vi "AnalogCNTL_Dakota2ch.vi"() -> ()   [LabVIEW 2015]
uses:
  <userlib>/caLab/Private/Put_DBL-1D_PV-1D.vi
  <vilib>/addons/control/pid/pid.llb/PID (DBL).vi
  <userlib>/caLab/Private/Get_PV-1D.vi
  <vilib>/addons/control/pid/NI_PID_pid.lvlib
  <vilib>/Analysis/NI_AALPro.lvlib
panel:
  out "slope OK":bool
  in  "slope loop":u8=15 min=10 max=30 step=1
  in  "Inlet2 offset":dbl
  out "APX:CellPressureState":u32
  in  "Threshold":dbl format="%#_13g"
  out "Inlet More":bool
  out "APX:OmniaxZ 2":dbl
  out "Open 2":bool
  in  "Gas_in_min_LIM 2":dbl min=0.0 max=0.3 step=0.02 format="%_3g"
  in  "Gas_in_max_LIM 2":dbl min=0.0 max=2.0 step=0.02 format="%_3g"
  out "Inlet2":dbl(slide) scale=0.3..0.8
  out "APX:CellIn2_Mv":dbl
  out "APX:CellOut_MV":dbl
  out "OmniazZ Failure":bool
  out "APX:CellMode":dbl
  out "APX:OmniaxZ":dbl
  out "APX:CellPressureState_LED":i16(slide) scale=0.0..3.0
  out "APX:CellPressureStateorg":i16
  out "APX:CellMode":bool
  out "PID_P":dbl format="%_4g"
  out "HPC Pressure Failure":bool
  out "HPC Turbo failure":bool
  out "<1.3":bool
  out "<2":bool
  out "APX:V7_SCL":bool
  out "APX:V7_SOP":bool
  out "OpenEx":bool
  out "APX:GAS":dbl format="%.2f"
  out "APX:CellIn_MV":dbl
  out "slope":dbl
  out "Open 1":bool
  in  "Inlet Mode":u16(ring) items=["Close", "Open", "Auto"]
  out "Inlet":sgl(slide)=0.8 min=0.3 max=0.8 step=0.05 scale=0.3..0.8
  out "Status":bool
  out "CellMode":u16
  out "Gas_out_max":dbl
  out "Period":i32
  out "Open Period":i32
  in  "Gas_in_min_LIM":dbl min=0.0 max=0.3 step=0.02 format="%_3g"
  in  "Gain":dbl=1.0 min=1.0 max=50.0 step=1.0 format="%_3g"
  in  "Gas_in_max_LIM":dbl=0.85 min=0.0 max=0.9 step=0.02 format="%_3g"
  in  "PID_D":dbl min=0.0 max=5.0 step=0.02 format="%_3g"
  in  "PID_I":dbl=0.5 min=0.005 max=5.0 step=0.02 format="%_3g"
  in  "PID_P_base":dbl=1.0 min=0.005 max=5.0 step=0.02 format="%_3g"
  in  "APX:CellPressure_RV":dbl=0.05 min=0.001 max=5.0 step=0.001 format="%.3f"
  out "PID_OC":dbl format="%.2f"
  out "PID dt out (s)":dbl format="%.3f"
  out "CellPressure":dbl(graph)
  in  "Exhasuet Mode":u16(ring) items=["Close", "Open", "Auto"]
  out "APX:AP1":dbl format="%#_3g"
  out "Outlet":sgl(slide)=2.0 min=0 max=5 step=0.05 scale=0.0..5.0
  out "APX:HPC":dbl format="%#_3g"
  out "APX:CellPressure_PV":dbl format="%_5g"
  in  "stop":bool
  # "Close-Close"
  # "Close-Open"
  # "Mk-II"
  # "0:Evacuate\n1: Auto-Auto\n2: Man-Man\n3: Man-Auto\n4: Auto-Man"
  # "Dakota 100000 sccm"
  # "if P>0.1 Period=Px100"
  # "8E-7 torr"
  # "record(ao, \"APX:CellIn_RV\")\n{\n    field(DESC, \"Double input without range infos\")\n    field(EGU, \"NA\")\n    field(PINI, \"YES\")\n}\nrecord(ao, \"APX:CellOut_RV\")\n{\n    field(DESC, \"Double input without range infos\")\n    field(EGU, \"NA\")\n    field(PINI, \"YES\")\n}\nrecord(ao, \"APX:CellIn_MV\")\n{\n    field(DESC, \"Double input without range infos\")\n    field(EGU, \"NA\")\n    field(PINI, \"YES\")\n}\nrecord(ao, \"APX:CellOut_MV\")\n{\n    field(DESC, \"Double input without range infos\")\n    field(EGU, \"NA\")\n    field(PINI, \"YES\")"
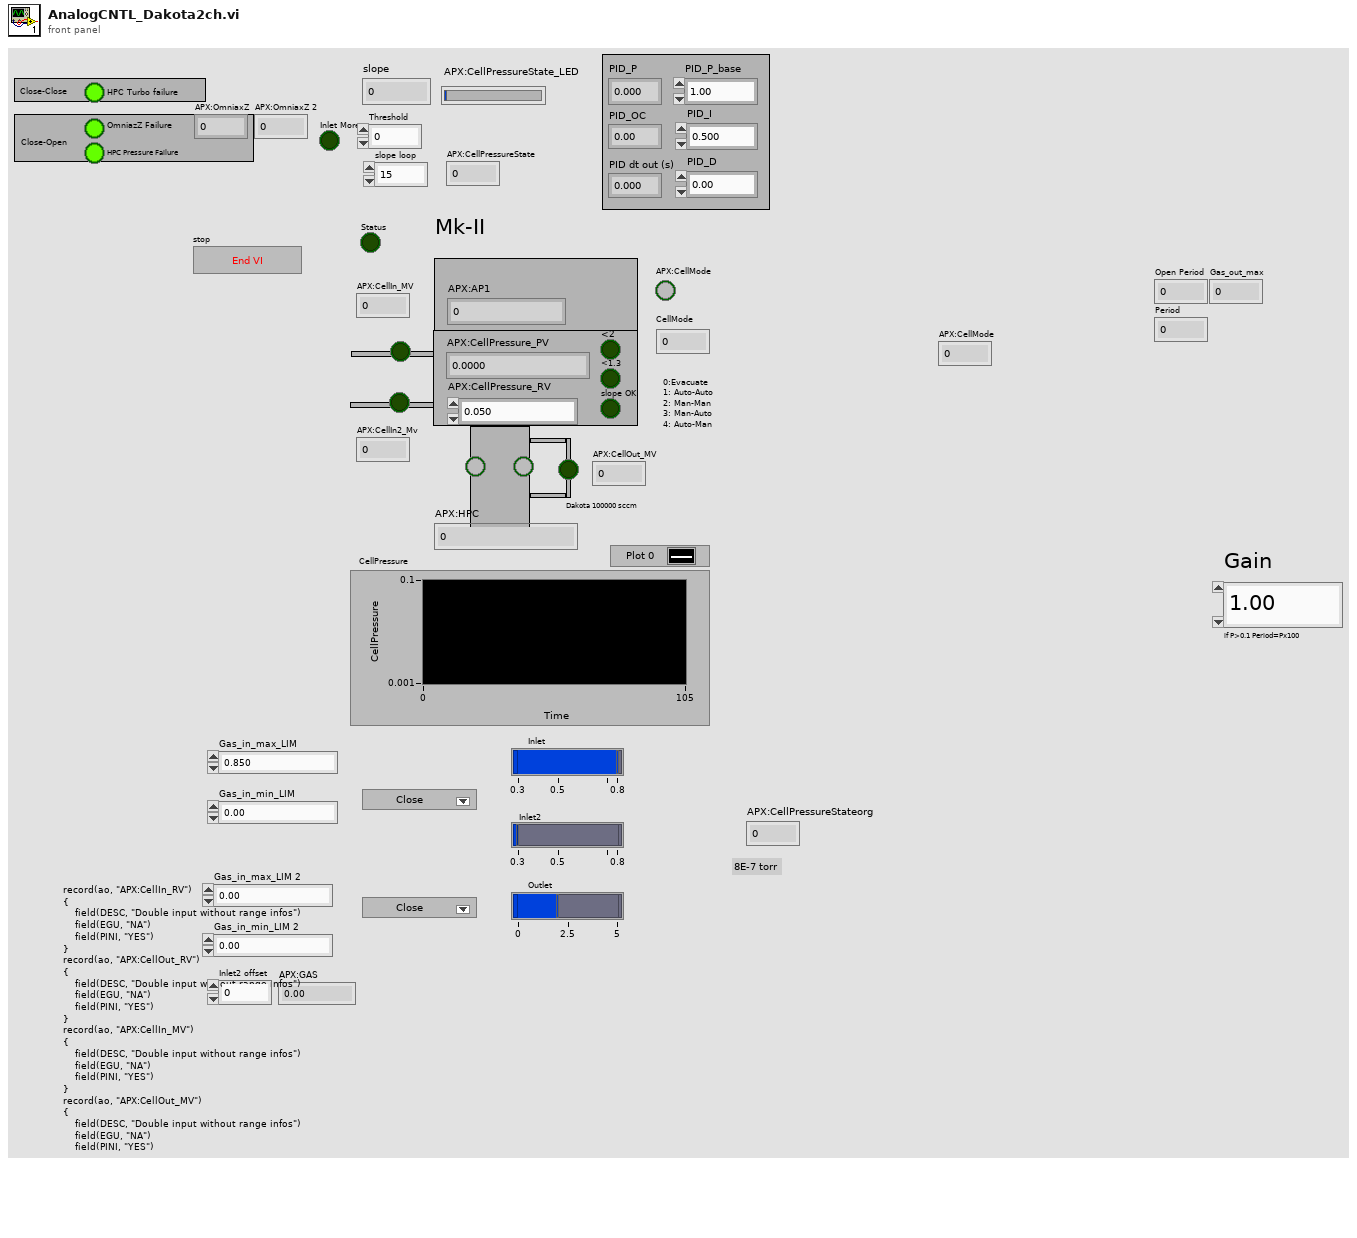
[diagram p1: front panel]
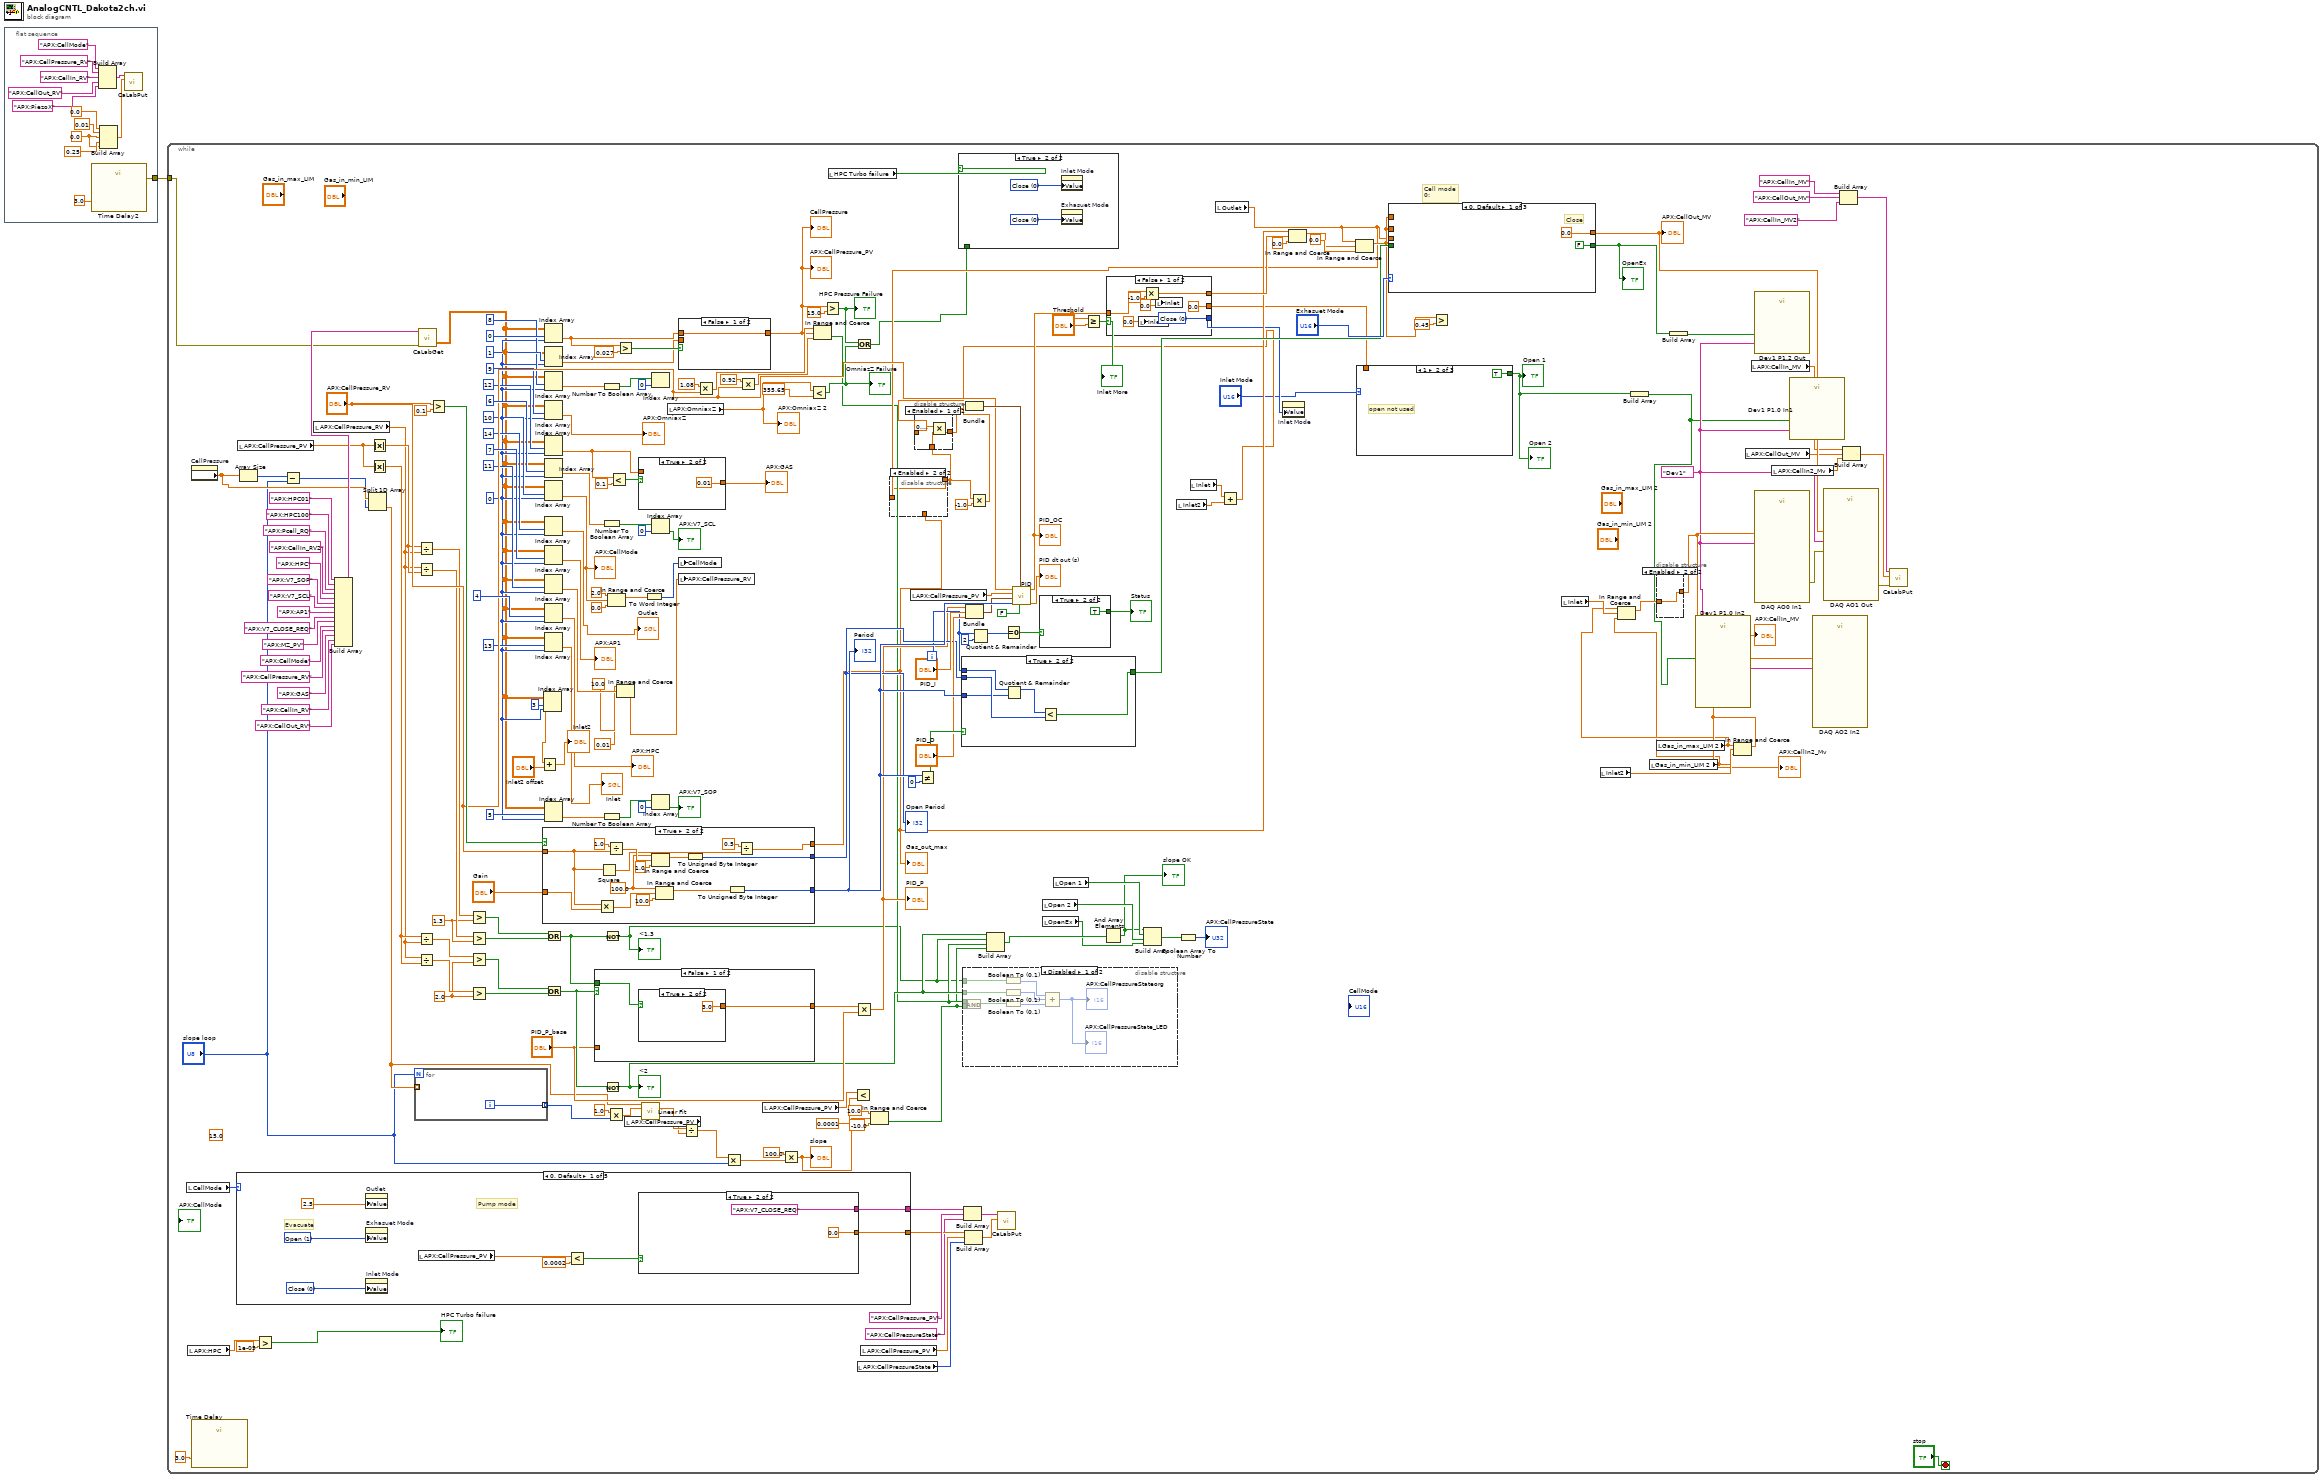
[diagram p0: block diagram]
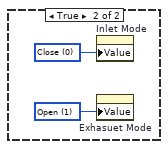
[diagram p8: hidden frame]
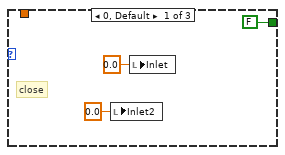
[diagram p9: hidden frame]
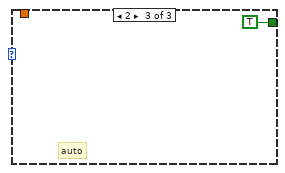
[diagram p10: hidden frame]
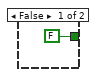
[diagram p11: hidden frame]
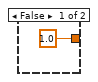
[diagram p12: hidden frame]
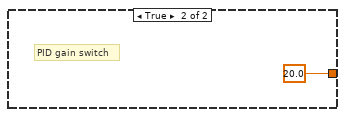
[diagram p13: hidden frame]
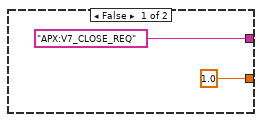
[diagram p14: hidden frame]
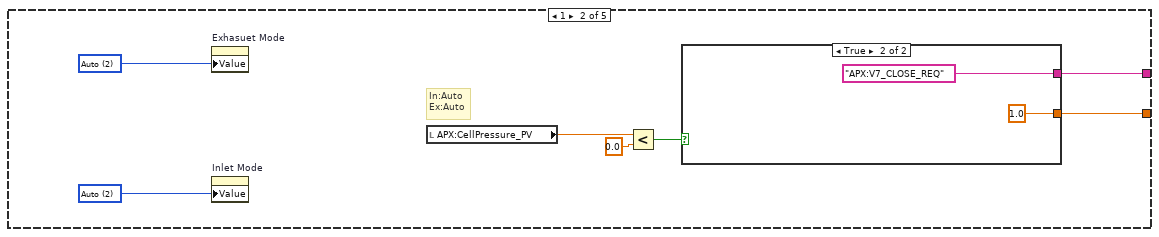
[diagram p15: hidden frame]
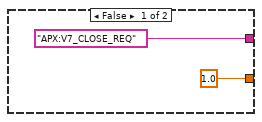
[diagram p16: hidden frame]
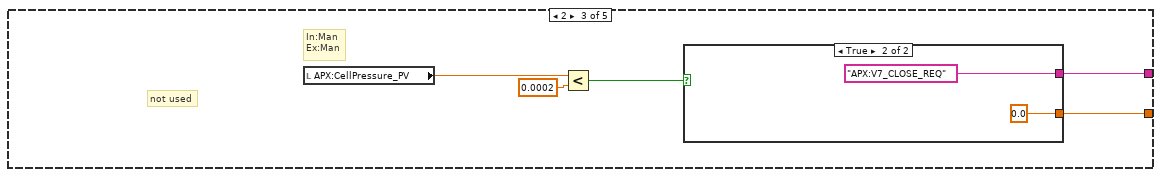
[diagram p17: hidden frame]
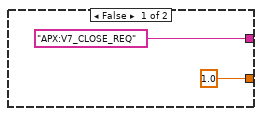
[diagram p18: hidden frame]
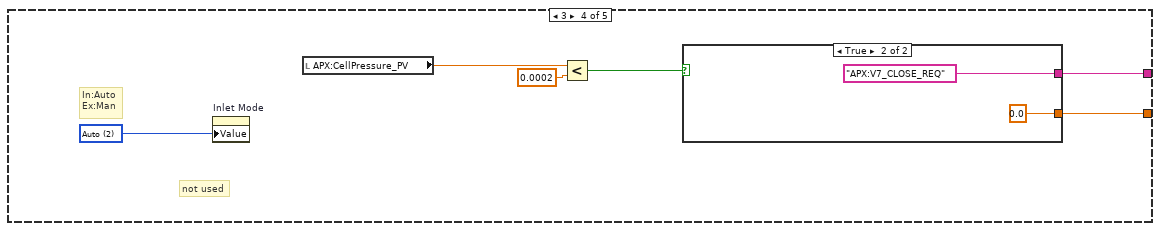
[diagram p19: hidden frame]
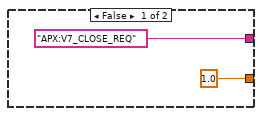
[diagram p20: hidden frame]
diagram:
  n1 = flat-sequence {
    tunnel: [w8] -> w1
    frame #0 {
      w2 = 0.0 ("element")
      n2 = call "Time Delay2"("Delay Time (s)"=3.0) -> ("error out"=w8:errorcluster)  [unwired: 10 in]
      n3 = Build Array("APX:CellMode", "APX:CellPressure_RV", "APX:CellIn_RV", "APX:CellOut_RV", "APX:PiezoX") -> (w12:string[])
      n4 = Build Array(0.0 ("element"), 0.01 ("element"), w2, 0.25 ("element"), w2) -> (w10:dbl[])
      n5 = call-poly <userlib>:"CaLabPut.vi"("Values"=w10, "PV Names"=w12) -> ()  [unwired: 6 in, 4 out]
    }
  }
  n6 = while {
    tunnel: w1 -> [w102]
    i -> [w157]
    stop <- "stop" stop-if-true
    w130 = 1.3 ("y")
    w139 = 2.0 ("y")
    (unwired) 15.0 ("y")
    w61 = 0 ("index (col)")
    w57 = tag "Dev1" ("device name")
    # "Cell mode \n0:"
    n7 = local read "CellMode"() -> (w92:u16)
    n8 = local read "APX:HPC"() -> (w120:dbl)
    n9 = property on="CellPressure" class="WFChart (strict)"() -> ("History Data"=w152:dbl[])  [unwired: 2 in, 2 out]
    n10 = call "Time Delay"("Delay Time (s)"=3.0) -> ()  [unwired: 10 in, 1 out]
    n11 = case shown="0, Default" w92 {
      tunnel: [w264 w275 w284 w294 w304] -> w108
      tunnel: [w263 w274 w283 w293 w303] -> w107
      frame 0, Default {
        w261 = u16 1 items=["Close", "Open", "Auto"] ("Exhasuet Mode")
        w262 = u16 0 items=["Close", "Open", "Auto"] ("Inlet Mod")
        # "Pump mode"
        # "Evacuate"
        n12 = property on="Outlet" class="Slide (strict)"("Value"=sgl 2.5 ("Exhaust")) -> ()  [unwired: 2 in, 2 out]
        n13 = property on="Exhasuet Mode" class="Ring (strict)"("Value"=w261) -> ()  [unwired: 2 in, 2 out]
        n14 = property on="Inlet Mode" class="Ring (strict)"("Value"=w262) -> ()  [unwired: 2 in, 2 out]
        n15 = local read "APX:CellPressure_PV"() -> (w259:dbl)
        n16 = Less?(x=w259, y=0.0002) -> (x < y?=w265:bool)
        n17 = case shown="True" w265 {
          tunnel: ["APX:V7_CLOSE_REQ" ("PV Name") "APX:V7_CLOSE_REQ" ("PV Name")] -> w264
          tunnel: [1.0 ("Value") 0.0 ("Value")] -> w263
          frame False {
          }
          frame True {
          }
        }
      }
      frame 1 {
        w272 = u16 2 items=["Close", "Open", "Auto"] ("Inlet Mod")
        w273 = u16 2 items=["Close", "Open", "Auto"] ("Exhasuet Mode")
        # "In:Auto\nEx:Auto"
        n18 = property on="Exhasuet Mode" class="Ring (strict)"("Value"=w273) -> ()  [unwired: 2 in, 2 out]
        n19 = property on="Inlet Mode" class="Ring (strict)"("Value"=w272) -> ()  [unwired: 2 in, 2 out]
        n20 = local read "APX:CellPressure_PV"() -> (w271:dbl)
        n21 = Less?(x=w271, y=0.0) -> (x < y?=w276:bool)
        n22 = case shown="True" w276 {
          tunnel: ["APX:V7_CLOSE_REQ" ("PV Name") "APX:V7_CLOSE_REQ" ("PV Name")] -> w275
          tunnel: [1.0 ("Value") 1.0 ("Value")] -> w274
          frame False {
          }
          frame True {
          }
        }
      }
      frame 2 {
        # "not used"
        # "In:Man\nEx:Man"
        n23 = local read "APX:CellPressure_PV"() -> (w282:dbl)
        n24 = Less?(x=w282, y=0.0002) -> (x < y?=w285:bool)
        n25 = case shown="True" w285 {
          tunnel: ["APX:V7_CLOSE_REQ" ("PV Name") "APX:V7_CLOSE_REQ" ("PV Name")] -> w284
          tunnel: [1.0 ("Value") 0.0 ("Value")] -> w283
          frame False {
          }
          frame True {
          }
        }
      }
      frame 3 {
        w292 = u16 2 items=["Close", "Open", "Auto"] ("Exhasuet Mode")
        # "not used"
        # "In:Auto\nEx:Man"
        n26 = property on="Inlet Mode" class="Ring (strict)"("Value"=w292) -> ()  [unwired: 2 in, 2 out]
        n27 = local read "APX:CellPressure_PV"() -> (w291:dbl)
        n28 = Less?(x=w291, y=0.0002) -> (x < y?=w295:bool)
        n29 = case shown="True" w295 {
          tunnel: ["APX:V7_CLOSE_REQ" ("PV Name") "APX:V7_CLOSE_REQ" ("PV Name")] -> w294
          tunnel: [1.0 ("Value") 0.0 ("Value")] -> w293
          frame False {
          }
          frame True {
          }
        }
      }
      frame 4 {
        w302 = u16 2 items=["Close", "Open", "Auto"] ("Exhasuet Mode")
        # "not used"
        # "In:Exhaust\nEx:Auto"
        n30 = property on="Exhasuet Mode" class="Ring (strict)"("Value"=w302) -> ()  [unwired: 2 in, 2 out]
        n31 = local read "APX:CellPressure_PV"() -> (w301:dbl)
        n32 = Less?(x=w301, y=0.0002) -> (x < y?=w305:bool)
        n33 = case shown="True" w305 {
          tunnel: ["APX:V7_CLOSE_REQ" ("PV Name") "APX:V7_CLOSE_REQ" ("PV Name")] -> w304
          tunnel: [1.0 ("Value") 0.0 ("Value")] -> w303
          frame False {
          }
          frame True {
          }
        }
      }
    }
    n34 = local read "APX:CellPressure_PV"() -> (w126:dbl)
    n35 = Array Size(array=w152) -> (size(s)=w150:i32)
    n36 = Greater?(x=w120, y=1e-05) -> (0:→"HPC Turbo failure":bool)
    n37 = Subtract(x=w150, y="slope loop") -> (x-y=w151:i32)
    n38 = local read "APX:CellPressure_RV"() -> (w125:dbl)
    n39 = Build Array("APX:HPC01", "APX:HPC100", "APX:Pcell_RQ", "APX:CellIn_RV2", "APX:HPC", "APX:V7_SOP", "APX:V7_SCL", "APX:AP1", "APX:V7_CLOSE_REQ", "APX:MZ_PV", "APX:CellMode", "APX:CellPressure_RV", "APX:GAS" ("element"), "APX:CellIn_RV", "APX:CellOut_RV") -> (w221:string[])
    n40 = Split 1D Array(array=w152, index=w151) -> (second subarray=w45:dbl[])  [unwired: 1 out]
    n41 = Absolute Value(x=w126) -> (abs(x)=w127:dbl)
    n42 = Absolute Value(x=w126) -> (abs(x)=w133:dbl)
    n43 = for {
      N: "slope loop" -> [_]
      tunnel: w45 -> [_] mode=indexing
      tunnel: [w246] -> w149 mode=indexing
      i -> [w246]
    }
    n44 = Divide(x=w127, y=w125) -> (x/y=w132:dbl)
    n45 = Divide(x=w125, y=w127) -> (x/y=w131:dbl)
    n46 = Divide(x=w133, y=w125) -> (x/y=w141:dbl)
    n47 = Divide(x=w125, y=w133) -> (x/y=w140:dbl)
    n48 = call-poly "CaLabGet.vi"("PV Names"=w221, "Error in (no error)"=w102) -> ("Value Array (number)"=w60:dbl[][])  [unwired: 7 in, 6 out]
    n49 = Greater?(x="APX:CellPressure_RV", y=0.1) -> (0:w189:bool)
    n50 = Greater?(x=w132, y=w130) -> (0:w129:bool)
    n51 = Greater?(x=w131, y=w130) -> (0:w128:bool)
    n52 = Greater?(x=w141, y=w139) -> (0:w138:bool)
    n53 = Greater?(x=w140, y=w139) -> (0:w137:bool)
    n54 = case shown="True" w189 {
      tunnel: "APX:CellPressure_RV" -> [_ w324]
      tunnel: [w322 w333] -> w188
      tunnel: "Gain" -> [_ w337]
      tunnel: [w322 w327] -> w169
      tunnel: [5.0 w325] -> w65
      frame False {
        w322 = 10
      }
      frame True {
        w330 = 100.0 ("upper limit")
        n55 = Multiply(x=w324, y=w337) -> (x*y=w335:dbl)
        n56 = Square(x=w324) -> (x^2=w323:dbl)
        n57 = Divide(x=1.0, y=w324) -> (x/y=w331:dbl)
        n58 = In Range and Coerce(upper limit=w330, x=w331, lower limit=1.0) -> (coerced(x)=w328:dbl)  [unwired: 1 out]
        n59 = In Range and Coerce(upper limit=w330, x=w335, lower limit=10.0) -> (coerced(x)=w334:dbl)  [unwired: 1 out]
        n60 = To Unsigned Byte Integer(number=w328) -> (unsigned 8bit integer=w327:u8)
        n61 = To Unsigned Byte Integer(number=w334) -> (unsigned 8bit integer=w333:u8)
        n62 = Divide(x=0.5, y=w323) -> (x/y=w325:dbl)
      }
    }
    "Open Period" <- w169
    "Period" <- w188
    "Gas_out_max" <- w65
    n63 = Index Array(array=w60, index (row)=3, index (col)=w61) -> (element=w21:dbl)
    n64 = Add(x=w21, y="Inlet2 offset") -> (x+y=→"Inlet2":dbl)
    n65 = Index Array(array=w60, index (row)=1 ("disabled index (col)"), index (col)=w61) -> (element=w215:dbl)
    n66 = Index Array(array=w60, index (row)=8, index (col)=w61) -> (element=w165:dbl)
    n67 = Index Array(array=w60, index (row)=9 ("disabled index (row)"), index (col)=w61) -> (element=→"APX:OmniaxZ":dbl)
    n68 = Index Array(array=w60, index (row)=6, index (col)=w61) -> (element=w203:dbl)
    n69 = Index Array(array=w60, index (row)=14 ("disabled index (row)"), index (col)=w61) -> (element=→"Outlet":dbl)
    n70 = Index Array(array=w60, index (row)=7, index (col)=w61) -> (element=→"APX:AP1":dbl)
    n71 = Index Array(array=w60, index (row)=11, index (col)=w61) -> (element=w100:dbl)
    n72 = Index Array(array=w60, index (row)=4, index (col)=w61) -> (element=→"APX:HPC":dbl)
    n73 = Index Array(array=w60, index (row)=13 ("disabled index (row)"), index (col)=w61) -> (element=→"Inlet":dbl)
    n74 = Index Array(array=w60, index (row)=5, index (col)=w61) -> (element=w202:dbl)
    n75 = Index Array(array=w60, index (row)=0 ("disabled index (col)"), index (col)=w61) -> (element=w214:dbl)
    n76 = Index Array(array=w60, index (row)=12, index (col)=w61) -> (element=w84:dbl)
    n77 = Index Array(array=w60, index (row)=10, index (col)=w61) -> (element=w91:dbl)
    "APX:CellMode" <- w91
    n78 = Or(x=w129, y=w128) -> (x .or. y?=w124:bool)
    n79 = Or(x=w138, y=w137) -> (x .or. y?=w136:bool)
    n80 = case shown="False" w136 {
      tunnel: "PID_P_base" -> [_ _]
      tunnel: w124 -> [w255 _]
      tunnel: [w254 20.0 ("y")] -> w121
      frame False {
        n81 = case shown="True" w255 {
          tunnel: [1.0 ("y") 3.0 ("y")] -> w254
          frame False {
          }
          frame True {
          }
        }
      }
      frame True {
        # "PID gain switch"
      }
    }
    n82 = Number To Boolean Array(number=w165) -> (Boolean array=w164:bool[])
    n83 = Number To Boolean Array(number=w203) -> (Boolean array=w201:bool[])
    n84 = Number To Boolean Array(number=w202) -> (Boolean array=w198:bool[])
    n85 = Not(x=w124) -> (.not. x?=w19:bool)
    "<1.3" <- w19
    n86 = Not(x=w136) -> (.not. x?=w31:bool)
    "<2" <- w31
    n87 = Multiply(x=1.0, y=w149) -> (x*y=w148:dbl[])
    n88 = In Range and Coerce(upper limit=2.0, x=w91, lower limit=0.0) -> (coerced(x)=w93:dbl)  [unwired: 1 out]
    n89 = Less?(x=w84, y=0.1) -> (x < y?=w85:bool)
    n90 = Greater?(x=w214, y=0.027) -> (0:w217:bool)
    n91 = In Range and Coerce(upper limit=10.0, x=w100, lower limit=0.01) -> (coerced(x)=w97:dbl)  [unwired: 1 out]
    n92 = local read "APX:CellPressure_PV"() -> (w43:dbl)
    n93 = case shown="True" w85 {
      tunnel: w84 -> [w239 _]
      tunnel: [w239 0.01] -> w83
      frame False {
      }
      frame True {
      }
    }
    "APX:GAS" <- w83
    n94 = call <vilib>:"Linear Fit.vi"("Y"=w45, "X"=w148) -> ("slope"=w153:dbl)  [unwired: 9 in, 4 out]
    n95 = To Word Integer(number=w93) -> (16bit integer=w94:i16)
    n96 = Index Array(array=w164, index=0) -> ()  [unwired: 1 out]
    n97 = Index Array(array=w201, index=0) -> (element=→"APX:V7_SCL":bool)
    n98 = Index Array(array=w198, index=0) -> (element=→"APX:V7_SOP":bool)
    n99 = local read "APX:OmniaxZ"() -> (w34:dbl)
    "APX:OmniaxZ 2" <- w34
    n100 = case shown="False" w217 {
      tunnel: w215 -> [_ w363]
      tunnel: [w362 w363] -> w116
      tunnel: w214 -> [w362 _]
      frame False {
      }
      frame True {
      }
    }
    "APX:CellPressure_PV" <- w116
    "CellPressure" <- w116
    n101 = local write "CellMode"(w94) -> ()
    n102 = local write "APX:CellPressure_RV"(w97) -> ()
    n103 = Divide(x=w153, y=w43) -> (x/y=w143:dbl)
    n104 = Multiply(x=1.08, y="APX:CellPressure_RV") -> (x*y=w175:dbl)
    n105 = Multiply(x=w143, y="slope loop") -> (x*y=w142:dbl)
    n106 = Multiply(x=0.92, y="APX:CellPressure_RV") -> (x*y=w176:dbl)
    n107 = local read "APX:CellPressure_PV"() -> (w134:dbl)
    n108 = Multiply(x=100.0, y=w142) -> (x*y=w146:dbl)
    "slope" <- w146
    n109 = Less?(x=w34, y=355.65) -> (x < y?=w33:bool)
    "OmniazZ Failure" <- w33
    n110 = In Range and Coerce(upper limit=w175, x=w116, lower limit=w176) -> (In Range?=w30:bool)  [unwired: 1 out]
    n111 = Greater?(x=w116, y=15.0) -> (0:w115:bool)
    "HPC Pressure Failure" <- w115
    n112 = local read "HPC Turbo failure"() -> (w37:bool)
    n113 = Less?(x=w134, y=0.0001) -> ()  [unwired: 1 out]
    n114 = Or(x=w115, y=w33) -> (x .or. y?=w36:bool)
    n115 = Multiply(x=w121, y="PID_P_base") -> (x*y=w123:dbl)
    "PID_P" <- w123
    n116 = local read "APX:CellPressureState"() -> (w89:u32)
    n117 = local read "APX:CellPressure_PV"() -> (w104:dbl)
    n118 = In Range and Coerce(upper limit=10.0, x=w146, lower limit=-10.0) -> (In Range?=w29:bool)  [unwired: 1 out]
    n119 = local read "APX:CellPressure_PV"() -> (w167:dbl)
    n120 = Not Equal?(x=w188, y=u8 0) -> (x != y?=w194:bool)
    n121 = case shown="True" w37 {
      tunnel: w36 -> [w241 _]
      frame False {
        n122 = case shown="False" w241 {
          frame False {
          }
          frame True {
            w242 = u16 1 items=["Close", "Open", "Auto"] ("Inlet Mod")
            w243 = u16 0 items=["Close", "Open", "Auto"] ("Exhasuet Mode")
            n123 = property on="Inlet Mode" class="Ring (strict)"("Value"=w243) -> ()  [unwired: 2 in, 2 out]
            n124 = property on="Exhasuet Mode" class="Ring (strict)"("Value"=w242) -> ()  [unwired: 2 in, 2 out]
          }
        }
      }
      frame True {
        w244 = u16 0 items=["Close", "Open", "Auto"] ("Inlet Mod")
        w245 = u16 0 items=["Close", "Open", "Auto"] ("Exhasuet Mode")
        n125 = property on="Inlet Mode" class="Ring (strict)"("Value"=w245) -> ()  [unwired: 2 in, 2 out]
        n126 = property on="Exhasuet Mode" class="Ring (strict)"("Value"=w244) -> ()  [unwired: 2 in, 2 out]
      }
    }
    n127 = case shown="True" w194 {
      tunnel: w157 -> [_ w361]
      tunnel: [FALSE w360] -> w154
      tunnel: w188 -> [_ w357]
      tunnel: w169 -> [_ w359]
      frame False {
      }
      frame True {
        n128 = Quotient & Remainder(x=w361, y=w357) -> (x-y*floor(x/y)=w358:i32)  [unwired: 1 out]
        n129 = Less?(x=w358, y=w359) -> (x < y?=w360:bool)
      }
    }
    n130 = disable-structure shown="Disabled" {
      disable-tunnel: w31 -> [w227 _]
      disable-tunnel: w30 -> [w226 _]
      disable-tunnel: w29 -> [w225 _]
      disable-tunnel: w19 -> [w224 _]
      frame Disabled {
        n131 = And(x=w226, y=w225) -> (x .and. y?=w232:bool)
        n132 = Boolean To (0,1)(Boolean=w224) -> (0, 1=w229:i16)
        n133 = Boolean To (0,1)(Boolean=w227) -> (0, 1=w230:i16)
        n134 = Boolean To (0,1)(Boolean=w232) -> (0, 1=w231:i16)
        n135 = Compound Arithmetic op=ADD(w229, w230, w231) -> (→"APX:CellPressureStateorg" →"APX:CellPressureState_LED":i16)
      }
      frame Enabled {
      }
    }
    n136 = Build Array(w108, "APX:CellPressure_PV", "APX:CellPressureState") -> (w105:string[])
    n137 = Build Array(w107, w104, w89) -> (w106:dbl[])
    n138 = Bundle(w123, "PID_I"="PID_I", "PID_D"="PID_D") -> (w184:cluster{dbl, "PID_I":dbl, "PID_D":dbl})  [unwired: 1 in]
    n139 = Quotient & Remainder(x=w157, y=2) -> (x-y*floor(x/y)=w160:i32)  [unwired: 1 out]
    n140 = Build Array(w31, w19, w30, w29) -> (w28:bool[])
    n141 = call-poly <userlib>:"CaLabPut.vi"("Values"=w106, "PV Names"=w105) -> ()  [unwired: 6 in, 4 out]
    n142 = Equal To 0?(x=w160) -> (x = 0?=w161:bool)
    n143 = case shown="True" w161 {
      tunnel: [FALSE ("Status") TRUE ("Status")] -> w158
      frame False {
      }
      frame True {
      }
    }
    "Status" <- w158
    n144 = local read "Open 2"() -> (w26:bool)
    n145 = local read "OpenEx"() -> (w25:bool)
    n146 = local read "Open 1"() -> (w27:bool)
    n147 = And Array Elements(Boolean array=w28) -> (logical AND=w15:bool)
    "slope OK" <- w15
    n148 = Build Array(w15, w27, w26, w25) -> (w24:bool[])
    n149 = local read "Inlet2"() -> (w47:dbl)
    n150 = Boolean Array To Number(Boolean array=w24) -> (number=→"APX:CellPressureState":u32)
    n151 = local read "Inlet"() -> (w46:sgl)
    n152 = local read "Outlet"() -> (w42:sgl)
    n153 = disable-structure shown="Enabled" {
      disable-tunnel: w65 -> [w237 _]
      disable-tunnel: [w237 w238] -> w39
      disable-tunnel: w42 -> [_ w238]
      frame Disabled {
      }
      frame Enabled {
      }
    }
    n154 = Multiply(x=w39, y=-1.0) -> (x*y=w64:dbl)
    n155 = Add(x=w46, y=w47) -> (x+y=w41:dbl)
    n156 = disable-structure shown="Enabled" {
      disable-tunnel: w41 -> [_ _]
      disable-tunnel: [w234 _] -> w40
      disable-tunnel: w39 -> [w235 _]
      frame Enabled {
        n157 = Multiply(x=sgl 0.1, y=w235) -> (x*y=w234:sgl)
      }
      frame Disabled {
      }
    }
    n158 = Bundle(w64, w40) -> (w181:cluster{dbl, sgl})  [unwired: 1 in]
    n159 = call-poly <vilib>:"PID.vi"("reinitialize? (F)"=FALSE, "output range"=w181, "dt (s)"=w188, "PID gains"=w184, "process variable"=w167, "setpoint"="APX:CellPressure_RV") -> ("dt out (s)"=→"PID dt out (s)":dbl, "output"=w170:dbl)  [unwired: 4 in]
    "PID_OC" <- w170
    n160 = Greater Or Equal?(x=w170, y="Threshold") -> (x >= y?=w179:bool)
    "Inlet More" <- w179
    n161 = case shown="False" w179 {
      tunnel: [w316 0.0] -> w171
      tunnel: w170 -> [w317 w319]
      tunnel: [0.0 w319] -> w38
      tunnel: [w313 w318] -> w18
      frame False {
        w313 = u16 0 items=["Close", "Open", "Auto"] ("Inlet Mode")
        n162 = local write "Inlet2"(0.0 ("Inlet2")) -> ()
        n163 = Multiply(x=w317, y=-1.0) -> (x*y=w316:dbl)
        n164 = local write "Inlet"(sgl 0.0 ("Inlet")) -> ()
      }
      frame True {
        w318 = u16 2 items=["Close", "Open", "Auto"] ("Inlet Mode")
      }
    }
    n165 = property on="Inlet Mode" class="Ring (strict)"("Value"=w18) -> ()  [unwired: 2 in, 2 out]
    n166 = In Range and Coerce(upper limit=w65, x=w171, lower limit=0.0) -> (coerced(x)=w68:dbl)  [unwired: 1 out]
    n167 = In Range and Coerce(upper limit=w42, x=w68, lower limit=0.0) -> (coerced(x)=w67:dbl)  [unwired: 1 out]
    n168 = case shown="1" "Inlet Mode" {
      tunnel: [FALSE TRUE TRUE] -> w48
      tunnel: w38 -> [_ _ _]
      frame 0, Default {
        # "close"
        n169 = local write "Inlet2"(0.0 ("Inlet2")) -> ()
        n170 = local write "Inlet"(sgl 0.0 ("Inlet")) -> ()
      }
      frame 1 {
        # "open not used"
      }
      frame 2 {
        # "auto"
      }
    }
    "Open 1" <- w48
    "Open 2" <- w48
    n171 = case shown="0, Default" "Exhasuet Mode" {
      tunnel: w154 -> [_ w343 w349]
      tunnel: [0.0 2.5 ("y") w353] -> w156
      tunnel: w67 -> [_ _ w353]
      tunnel: w67 -> [_ _ w352]
      tunnel: w42 -> [_ w341 _]
      tunnel: [FALSE w342 w348] -> w70
      frame 0, Default {
        # "Close"
      }
      frame 1 {
        # "open"
        n172 = Equal?(x=w341, y=0.0) -> (x = y?=w344:bool)
        n173 = case shown="True" w344 {
          tunnel: w343 -> [_ _]
          tunnel: [TRUE TRUE] -> w342
          frame False {
          }
          frame True {
          }
        }
      }
      frame 2 {
        # "auto"
        n174 = Equal?(x=w352, y=0.0) -> (x = y?=w350:bool)
        n175 = case shown="True" w350 {
          tunnel: w349 -> [w354 _]
          tunnel: [w354 FALSE] -> w348
          frame False {
          }
          frame True {
            (unwired) 0.0
          }
        }
      }
    }
    "OpenEx" <- w70
    "APX:CellOut_MV" <- w156
    n176 = Greater?(x=w67, y=0.45) -> ()  [unwired: 1 out]
    n177 = local read "Inlet"() -> (w56:sgl)
    n178 = local read "Inlet2"() -> (w54:dbl)
    n179 = Build Array(w48) -> (w32:bool[])
    n180 = local read "Gas_in_min_LIM 2"() -> (w51:dbl)
    n181 = local read "Gas_in_max_LIM 2"() -> (w52:dbl)
    n182 = In Range and Coerce(upper limit=w52, x=w56, lower limit=w51) -> (coerced(x)=w55:dbl)  [unwired: 1 out]
    n183 = disable-structure shown="Enabled" {
      disable-tunnel: [_ w236] -> w63
      disable-tunnel: w55 -> [_ w236]
      frame Disabled {
      }
      frame Enabled {
      }
    }
    "APX:CellIn_MV" <- w63
    n184 = Build Array(w70) -> (w155:bool[])
    n185 = call "Dev1 P1.0 In2"("data"=w32, "device name"=w57) -> ()  [unwired: 16 in, 2 out]
    n186 = In Range and Coerce(upper limit=w52, x=w54, lower limit=w51) -> (coerced(x)=w53:dbl)  [unwired: 1 out]
    "APX:CellIn2_Mv" <- w53
    n187 = local read "APX:CellOut_MV"() -> (w71:dbl)
    n188 = local read "APX:CellIn_MV"() -> (w72:dbl)
    n189 = call "Dev1 P1.2 Out"("data"=w155, "device name"=w57) -> ()  [unwired: 16 in, 2 out]
    n190 = call "DAQ AO0 In1"("data"=w63, "device name"=w57) -> ("error out"=w74:errorcluster)  [unwired: 16 in, 1 out]
    n191 = local read "APX:CellIn2_Mv"() -> (w49:dbl)
    n192 = call "Dev1 P1.0 In1"("data"=w32, "device name"=w57) -> ()  [unwired: 16 in, 2 out]
    n193 = call "DAQ AO2 In2"("data"=w53, "device name"=w57) -> ()  [unwired: 16 in, 2 out]
    n194 = call "DAQ AO1 Out"("data"=w156, "error in"=w74, "device name"=w57) -> ("error out"=w73:errorcluster)  [unwired: 15 in, 1 out]
    n195 = Build Array("APX:CellIn_MV", "APX:CellOut_MV", "APX:CellIn_MV2") -> (w76:string[])
    n196 = Build Array(w72, w71, w49) -> (w75:dbl[])
    n197 = call-poly <userlib>:"CaLabPut.vi"("Error in (no error)"=w73, "Values"=w75, "PV Names"=w76) -> ()  [unwired: 5 in, 4 out]
  }
